vi "保存数据消息.vi"(1 "COM":i32, 2 "A":i32) -> ()   [LabVIEW 2015]
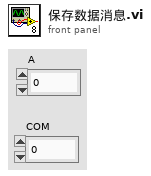
[diagram p1: front panel]
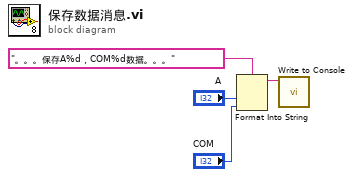
[diagram p0: block diagram]
diagram:
  n1 = Format Into String(format string="。。。保存A%d，COM%d数据。。。", "A", "COM") -> (resulting string=w1:string)  [unwired: 2 in, 1 out]
  n2 = call "Write to Console.vi"("Input"=w1) -> ()  [unwired: 10 in, 1 out]
